vi "multiPowSpect.vi"(6 "subLength":i32=2048, 7 "window":T1=1 items=["Rectangle"=0, "Hanning"=1, "Hamming"=2, "Blackman-Harris"=3, "Exact Blackman"=4, "Blackman"=5, "Flat Top"=6, "4 Term B-Harris "=7, "7 Term B-Harris"=8, "Low Sidelobe"=9, "Blackman Nuttall"=11, "Triangle"=30, "Bartlett-Hanning"=31, "Bohman"=32, "Parzen"=33, "Welch"=34, "Kaiser"=60, "Dolph-Chebyshev"=61, "Gaussian"=62], 8 "error in":errorcluster, 9 "overlap(0- 0.9)":dbl=0.5 min=0.0 max=0.9 step=0.1, 10 "timeseries":dbl[](array[numeric]) format="%_3e", 11 "samplingFrequency":dbl) -> (0 "error out":errorcluster, 2 "PSDdB":cluster{"f0":dbl, "df":dbl, "PSD(f)":dbl[]}, 4 "coresFFT":i32)   [LabVIEW 2022 SP3]
uses:
  <vilib>/Analysis/4window.llb/windowTd.ctl
  <vilib>/Analysis/baseanly.llb/Mean (DBL).vi
  <vilib>/Analysis/1siggen.llb/Ramp Pattern by Delta.vi
  <vilib>/Analysis/baseanly.llb/Std Deviation and Variance.vi
  <vilib>/Analysis/0measdsp.llb/Scaled Time Domain Window.vi
  <vilib>/Analysis/0measdsp.llb/Scaled Time Domain Window (DBL).vi
  <vilib>/Analysis/0measdsp.llb/Auto Power Spectrum.vi
  <vilib>/ErrorRing/Error Ring.xnode
  <vilib>/Analysis/NI_AALBase.lvlib
  <vilib>/Analysis/NI_AALPro.lvlib
panel:
  out "coresMean":i32
  out "nSpectra":i32
  out "shift":dbl
  out "PSD":cluster{dbl, "dF":dbl, dbl[]}(graph)
  out "newdF":dbl
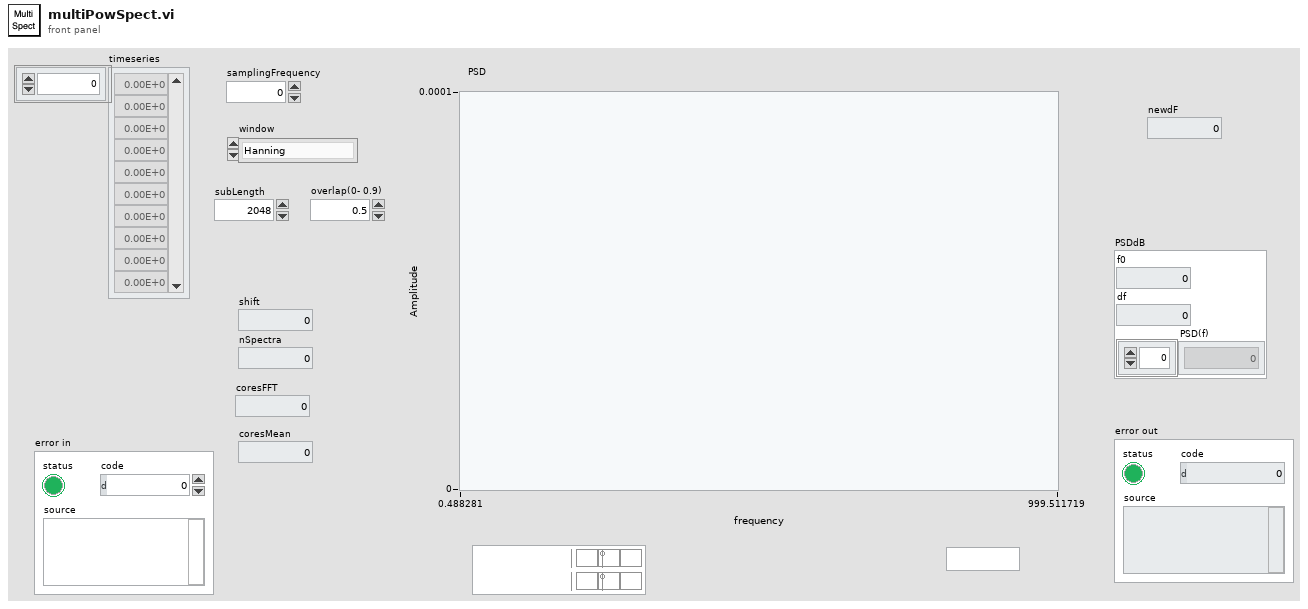
[diagram p1: front panel]
types:
  T1 = typedef "NI_AALPro.lvlib/windowTd.ctl" = u32
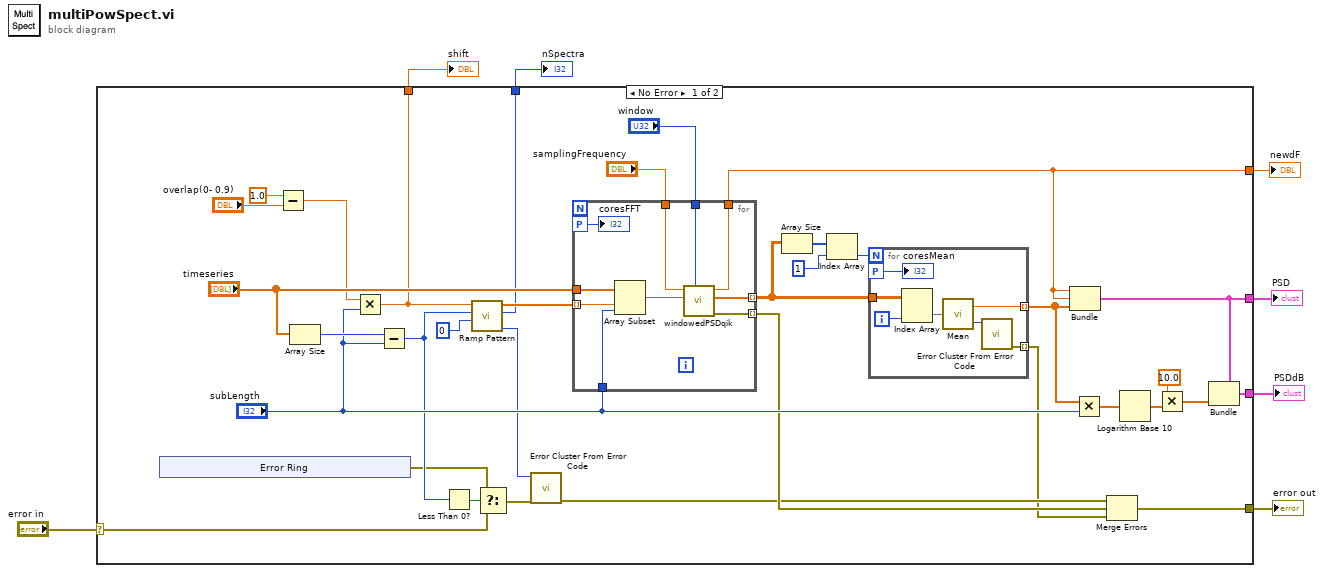
[diagram p0: block diagram]
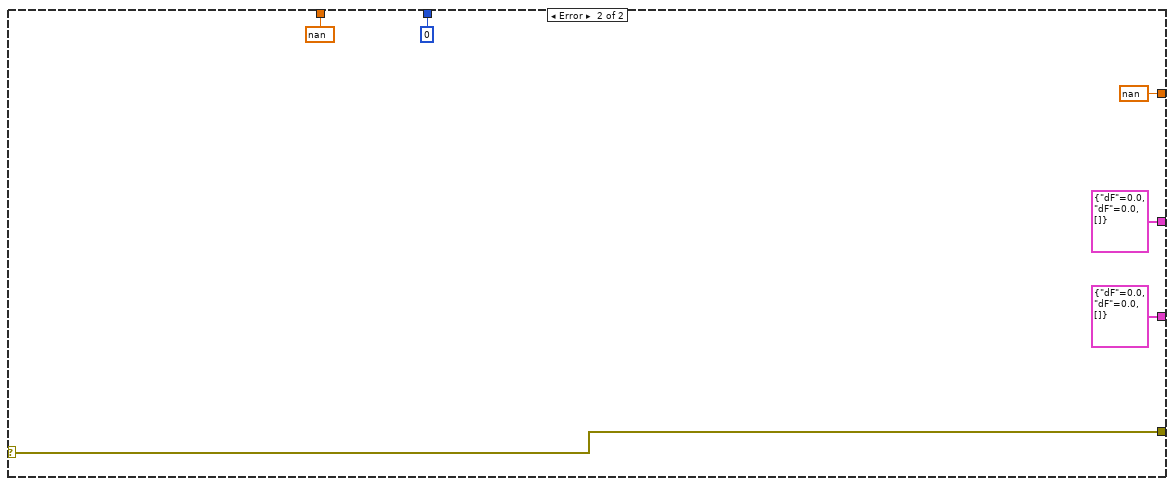
[diagram p2: hidden frame]
diagram:
  n1 = case shown="No Error" "error in" {
    selector: "error in" -> [w8 w69]
    tunnel: [w35 cluster{"dF":dbl, "dF":dbl, dbl[]} {"dF"=0.0, "dF"=0.0, []}] -> w7
    tunnel: [w33 cluster{"dF":dbl, "dF":dbl, dbl[]} {"dF"=0.0, "dF"=0.0, []}] -> w6
    tunnel: [w31 nan] -> w5
    tunnel: [w27 nan ("dF")] -> w4
    tunnel: [w22 0 ("samples")] -> w3
    tunnel: [w9 w69] -> w2
    frame No Error {
      n2 = xnode "Error Ring"() -> ("error out"=w14:errorcluster)
      n3 = Subtract(x=1.0, y="overlap(0- 0.9)") -> (x-y=w24:dbl)
      n4 = Array Size(array="timeseries") -> (size(s)=w29:i32)
      n5 = Multiply(x=w24, y="subLength") -> (x*y=w31:dbl)
      n6 = Subtract(x=w29, y="subLength") -> (x-y=w17:i32)
      n7 = Less Than 0?(x=w17) -> (x < 0?=w15:bool)
      n8 = call-poly <vilib>:"Ramp Pattern.vi"("start"=0, "end"=w17, "delta"=w31) -> ("error"=w16:i32, "samples"=w22:i32, "Ramp Pattern"=w32:dbl[])  [unwired: 6 in]
      n9 = Select(t=w14, s=w15, f=w8) -> (s? t:f=w13:errorcluster)
      n10 = call <vilib>:"Error Cluster From Error Code.vi"("error in (no error)"=w13, "error code (0)"=w16) -> ("error out"=w11:errorcluster)  [unwired: 7 in]
      n11 = for {
        tunnel: "timeseries" -> [w63]
        tunnel: "subLength" -> [w57]
        tunnel: "samplingFrequency" -> [w61]
        tunnel: [w60] -> w27
        tunnel: "window" -> [w59]
        tunnel: [w58] -> w21 mode=indexing
        workers-P: _ -> [w55]
        tunnel: w32 -> [w56] mode=indexing
        tunnel: [w54] -> w12 mode=indexing
        n12 = Array Subset(array=w63, index=w56, length=w57) -> (w62:dbl[])
        n13 = call "windowedPSDqik.vi"("window"=w59, "x(t)"=w62, "Fs"=w61) -> ("error out"=w54:errorcluster, "PSD(f)noDC"=w58:dbl[], "dF"=w60:dbl)  [unwired: 4 in, 2 out]
        "coresFFT" <- w55
      }
      n14 = Array Size(array=w21) -> (size(s)=w20:i32[])
      n15 = Index Array(array=w20, index=1) -> (element=w19:i32)
      n16 = for {
        N: w19 -> [_]
        tunnel: w21 -> [w53]
        tunnel: [w52] -> w26 mode=indexing
        workers-P: _ -> [w49]
        tunnel: [w47] -> w10 mode=indexing
        i -> [w50]
        n17 = Index Array(array=w53, index (col)=w50) -> (element=w51:dbl[])  [unwired: 1 in]
        n18 = call-poly <vilib>:"Mean.vi"("X"=w51) -> ("mean"=w52:dbl, "error"=w48:i32)
        n19 = call <vilib>:"Error Cluster From Error Code.vi"("error code (0)"=w48) -> ("error out"=w47:errorcluster)  [unwired: 8 in]
        "coresMean" <- w49
      }
      n20 = Bundle("dF"=w27, "dF"=w27, w26) -> (w35:cluster{"dF":dbl, "dF":dbl, dbl[]})  [unwired: 1 in]
      n21 = Multiply(x=w26, y="subLength") -> (x*y=w38:dbl[])
      n22 = Merge Errors(w11, w12, w10) -> (w9:errorcluster)
      n23 = Logarithm Base 10(1:w38) -> (0:w40:dbl[])
      n24 = Multiply(x=10.0, y=w40) -> (x*y=w34:dbl[])
      n25 = Bundle(cluster=w35, w34) -> (w33:cluster{"dF":dbl, "dF":dbl, dbl[]})  [unwired: 2 in]
    }
    frame Error {
    }
  }
  "newdF" <- w4
  "PSD" <- w7
  "PSDdB" <- w6
  "shift" <- w5
  "nSpectra" <- w3
  "error out" <- w2
